vi "Autoscan_EmitterReportGeneration.vi"(6 "Numeric":i32, 9 "Map centers short":dbl[](array[numeric]), 10 "reference in":refnum<vi>, 11 "Path in":refnum<vi>) -> (1 "String":string, 2 "appended path":path, 3 "appended path 2":path)   [LabVIEW 2023]
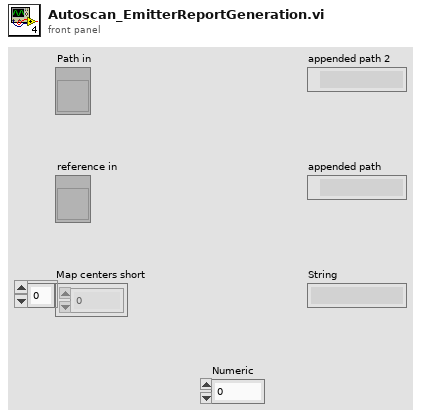
[diagram p1: front panel]
diagram:
  # "PI Stage"
  # "TCSPC"
  n1 = Index Array(array="Map centers short", index=0) -> (element=w17:dbl)
  n2 = property class="Path"(reference="Path in") -> ("Value"=w11:path)  [unwired: 1 in, 2 out]
  n3 = property class="Path"(reference="Path in") -> ("Value"=w3:path)  [unwired: 1 in, 2 out]
  n4 = Index Array(array="Map centers short", index=1) -> (element=w19:dbl)
  n5 = Multiply(x=w17, y=100) -> (x*y=w20:dbl)
  n6 = Add(x=w20, y=w19) -> (x+y=w21:dbl)
  n7 = Increment(x="Numeric") -> (x+1=w13:i32)
  n8 = To Word Integer(number=w21) -> (16bit integer=w22:i16)
  n9 = property class="DigNum (strict)"(reference="reference in", "Value"=w22) -> ()  [unwired: 1 in, 2 out]
  n10 = call "AUTOFLIM_Create_Filename.vi"("Y"=-1.0, "Term"=".csv", "Emitter #"=w13, "String"="Emitter report Area #", "start path"=w11) -> ("appended path"=→"appended path 2":path)  [unwired: 6 in]
  n11 = call "AUTOFLIM_Create_Filename.vi"("X"=-1.0, "Y"=-1.0, "Term"=".jpg", "Emitter #"=w13, "String"="PL map Area #", "start path"=w3) -> ("appended path"=w24:path)  [unwired: 5 in]
  "appended path" <- w24
  n12 = Path To String(path=w24) -> (string=→"String":string)
